vi "Crossmatch_and_Populate_Sick_Array.vi"(10 "Array":dbl[](array[numeric])) -> ()   [LabVIEW 2009]
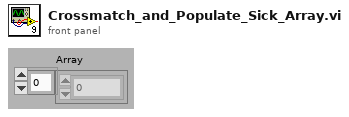
[diagram p1: front panel]
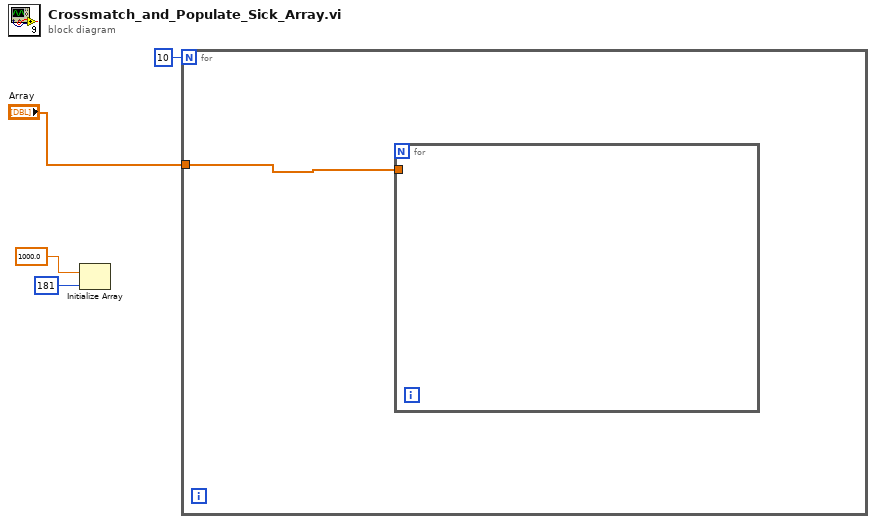
[diagram p0: block diagram]
diagram:
  n1 = Initialize Array(1000.0 ("element"), 181 ("dimension size")) -> ()  [unwired: 1 out]
  n2 = for {
    N: 10 -> [_]
    tunnel: "Array" -> [w5]
    i -> [w6]
    n3 = for {
      tunnel: w5 -> [_]
    }
  }
